vi "Create Sensor Menu.vi"(7 "beforeMenuItemID":i32, 8 "error in (no error)":errorcluster caption="错误输入（无错误）", 9 "beforeMenuID":i32, 10 "menuBarHandle":i32, 11 "sensorHandle":i32) -> (0 "error out":errorcluster caption="错误输出", 3 "function return":i32)   [LabVIEW 2018]
doc: "extern int __stdcall APSxCreateSensorMenu (int sensorHandle, IN int menuBarHandle, IN int beforeMenuID, IN int beforeMenuItemID);"
uses:
  APSx.dll/APSx.dll
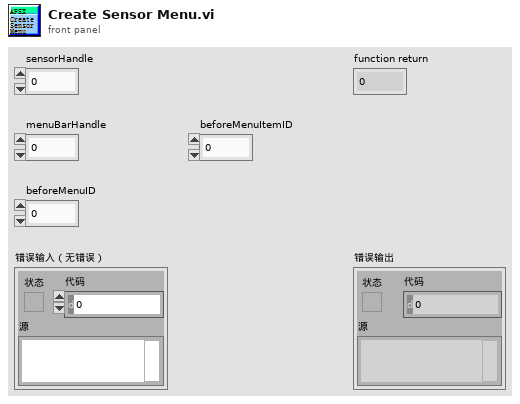
[diagram p1: front panel]
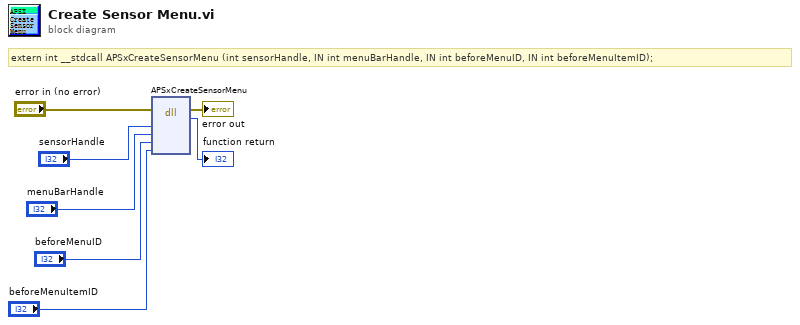
[diagram p0: block diagram]
diagram:
  # "extern int __stdcall APSxCreateSensorMenu (int sensorHandle, IN int menuBarHandle, IN int beforeMenuID, IN int beforeMenuItemID);"
  n1 = dll-call lib="PTH2[abs D项目Feng恒隆项目Labview传感器对中台SourcesAPSx.dllAPSx.*" fn="APSxCreateSensorMenu"(error in="error in (no error)", "sensorHandle"="sensorHandle", "menuBarHandle"="menuBarHandle", "beforeMenuID"="beforeMenuID", "beforeMenuItemID"="beforeMenuItemID") -> (error out=→"error out":errorcluster, →"function return":i32)  [unwired: 6 in, 1 out]
